vi "Set_Target_Duration.vi"(8 "error in (no error)":errorcluster, 10 "Elevator in":T2, 11 "Elevator Fleet in":T1) -> (0 "error out":errorcluster, 1 "Target Duration":dbl, 2 "Elevator out":T2, 3 "Elevator Fleet out":T1)   [LabVIEW 2026]
uses:
  Controls/Occupy_Status.ctl
  Controls/Door_Status_Enum.ctl
  Controls/Floor_Status.ctl
  Controls/Motion_Status_Enum.ctl
  Controls/Car_Calls_Status.ctl
  Controls/Hall_Calls_Status.ctl
  Controls/Elevator_Status.ctl
  Controls/Elevator_Fleet.ctl
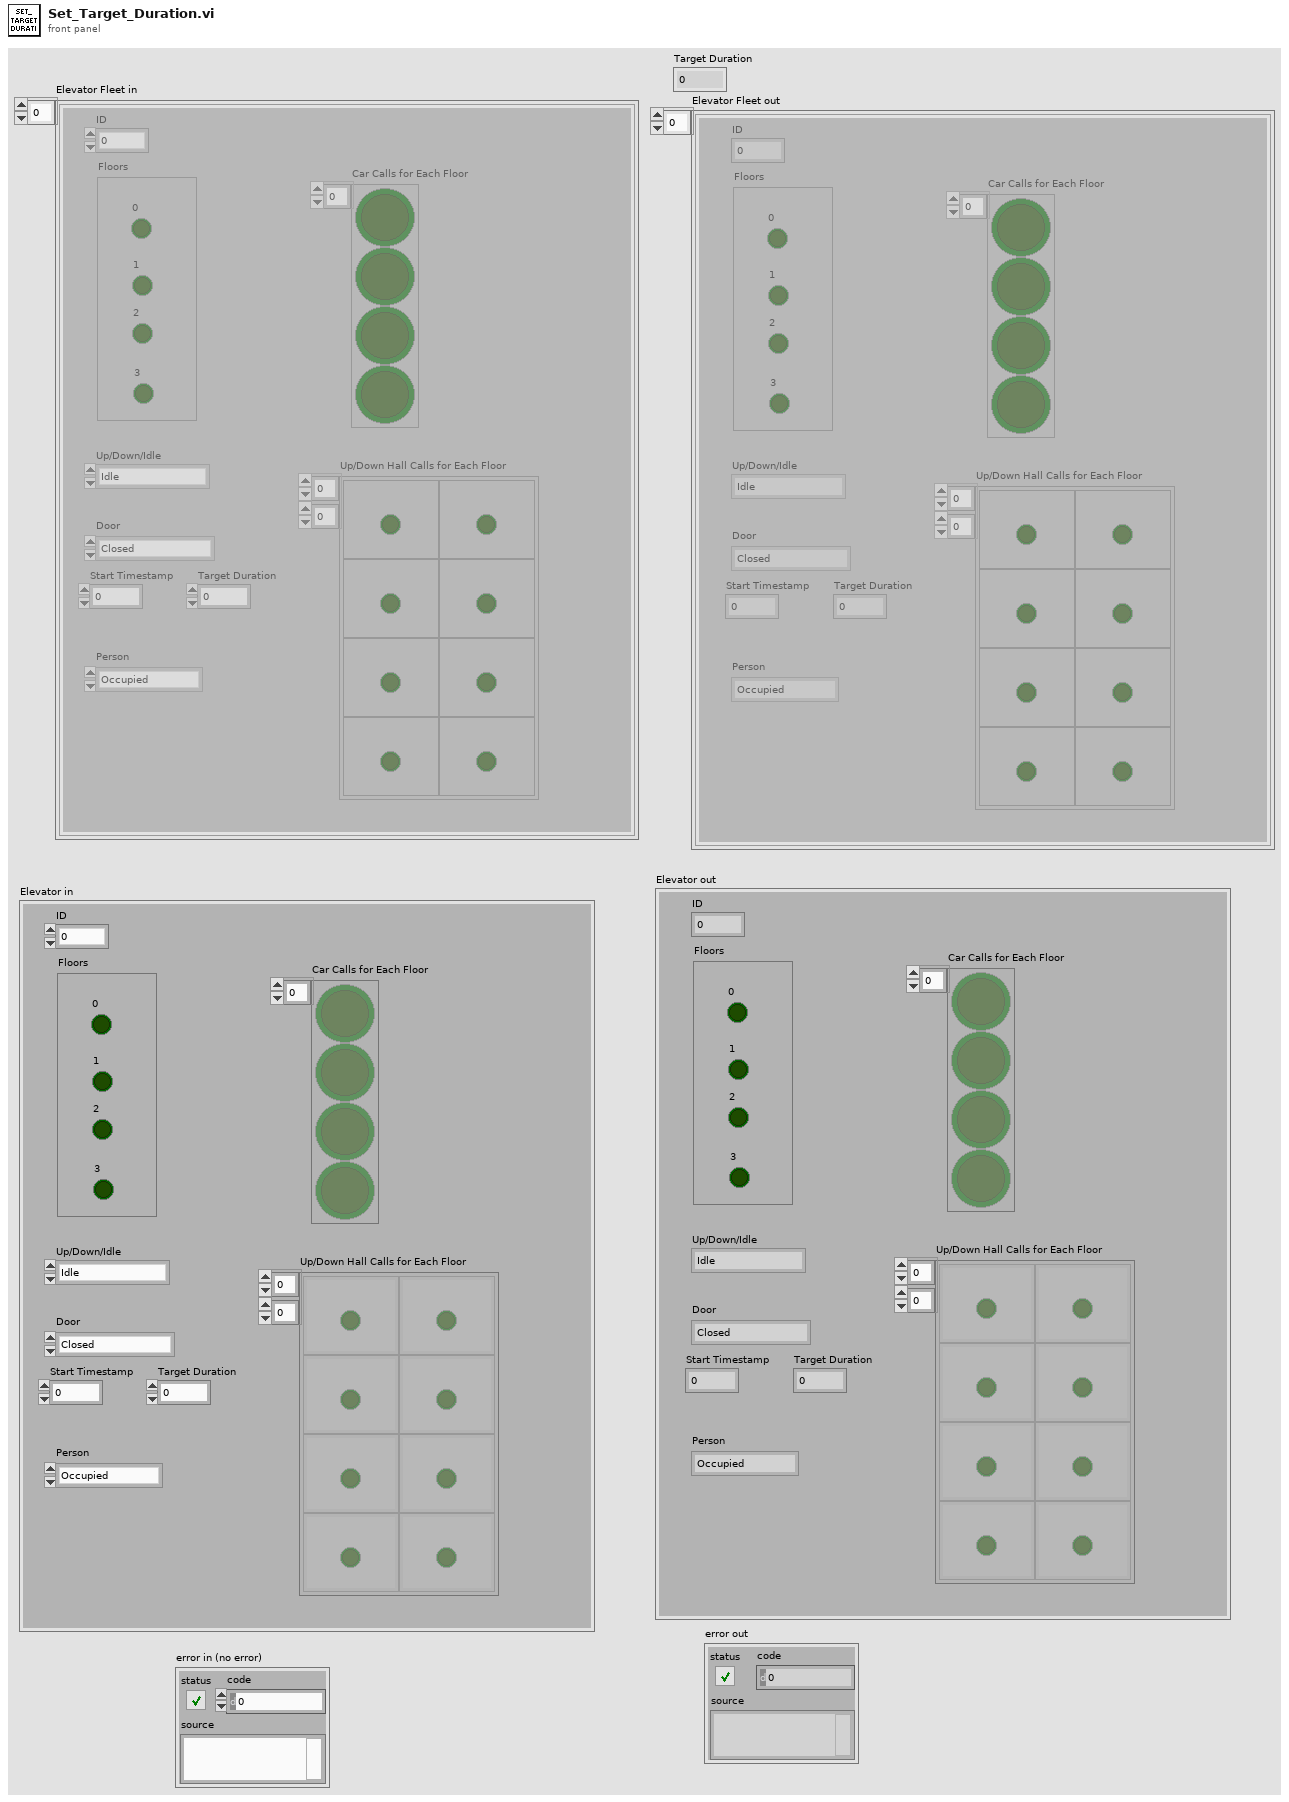
[diagram p1: front panel]
types:
  T1 = typedef "Elevator_Fleet.ctl" = T2[]
  T2 = typedef "Elevator_Status.ctl" = cluster{"Door":T3, "Person":T4, "Floors":T5, "Up/Down/Idle":T6, "Car Calls for Each Floor":T7, "Up/Down Hall Calls for Each Floor":T8, "ID":i32, "Start Timestamp":u32, "Target Duration":dbl}
  T3 = typedef "Door_Status_Enum.ctl" = enum16{"Closed", "Open", "Opening", "Closing"}
  T4 = typedef "Occupy_Status.ctl" = enum16{"Occupied", "Empty"}
  T5 = typedef "Floor_Status.ctl" = cluster{"0":bool, "1":bool, "2":bool, "3":bool}
  T6 = typedef "Motion_Status_Enum.ctl" = enum16{"Idle", "Up", "Down"}
  T7 = typedef "Car_Calls_Status.ctl" = bool[]
  T8 = typedef "Hall_Calls_Status.ctl" = cluster{bool}[][]
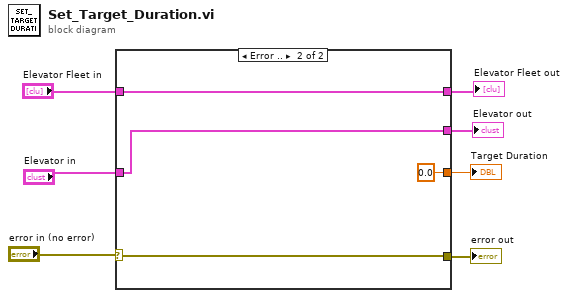
[diagram p0: block diagram]
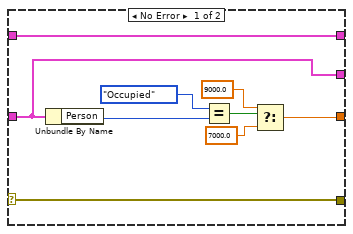
[diagram p2: hidden frame]
diagram:
  n1 = case shown="Error .." "error in (no error)" {
    selector: "error in (no error)" -> [w10 w17]
    tunnel: [w16 0.0 ("t")] -> w7
    tunnel: "Elevator in" -> [w8 w19]
    tunnel: [w10 w17] -> w4
    tunnel: "Elevator Fleet in" -> [w9 w20]
    tunnel: [w9 w20] -> w2
    tunnel: [w8 w19] -> w1
    frame No Error {
      n2 = Unbundle By Name(w8) -> ("Person"=w11:T4)
      n3 = Equal?(x=Occupy_Status."Occupied", y=w11) -> (x = y?=w13:bool)
      n4 = Select(t=9000.0, s=w13, f=7000.0 ("t")) -> (s? t:f=w16:dbl)
    }
    frame Error {
    }
  }
  "Target Duration" <- w7
  "error out" <- w4
  "Elevator out" <- w1
  "Elevator Fleet out" <- w2
